vi "NI USB GPIB Command.vi"(4 "close?":bool, 6 "initialize?":bool, 8 "Error In":errorcluster, 10 "write buffer":string="X", 11 "VISA resource name":refnum<visa-resource-name>="GPIB1::25::INSTR") -> (0 "Error Out":errorcluster, 2 "read buffer":string, 3 "VISA resource name out":refnum<visa-resource-name>)   [LabVIEW 2016, in "IPS-120.lvlib"]
uses:
  IPS-120.lvlib
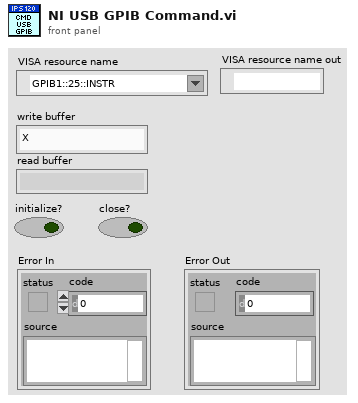
[diagram p1: front panel]
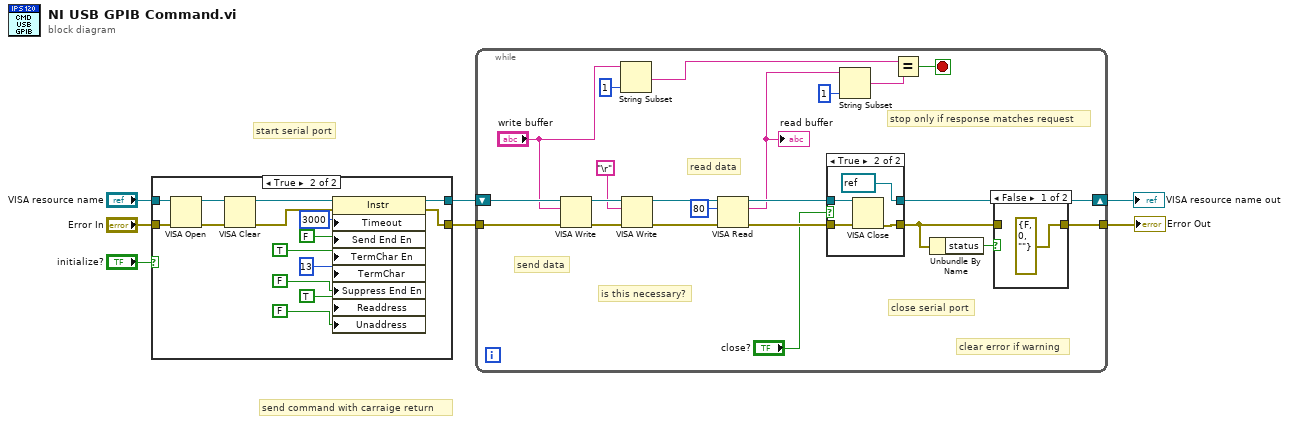
[diagram p0: block diagram]
diagram:
  # "send command with carraige return"
  # "start serial port"
  n1 = case shown="True" "initialize?" {
    tunnel: [w8 w16] -> w7
    tunnel: "Error In" -> [w9 w12]
    tunnel: [w9 w10] -> w4
    tunnel: "VISA resource name" -> [w8 w11]
    frame False {
    }
    frame True {
      n2 = VISA Open(error in (no error)=w12, VISA resource name=w11) -> (VISA resource name=w19:refnum<visa-resource-name>, error out=w20:errorcluster)  [unwired: 3 in]
      n3 = VISA Clear(VISA resource name=w19, error in (no error)=w20) -> (VISA resource name out=w17:refnum<visa-resource-name>, error out=w18:errorcluster)
      n4 = property class="Instr"(reference=w17, error in=w18, "Timeout"=u32 3000 ("General Settings:Timeout Value"), "Send End En"=FALSE ("Message Based Settings:Send End Enable"), "TermChar En"=TRUE ("Message Based Settings:Termination Character Enable"), "TermChar"=u8 13 ("Message Based Settings:Termination Character"), "Suppress End En"=FALSE ("Message Based Settings:Suppress End Enable"), "Readdress"=TRUE ("GPIB Settings:Readdressing"), "Unaddress"=FALSE ("GPIB Settings:Unaddressing")) -> (reference out=w16:refnum<visa-resource-name>, error out=w10:errorcluster)
    }
  }
  n5 = while {
    shift-right: [w28] -> w1
    shift-left: w7 -> [w42]
    tunnel: w4 -> [w34]
    tunnel: [w37] -> w6
    stop <- w25 stop-if-true
    # "stop only if response matches request"
    # "clear error if warning"
    # "is this necessary?"
    # "send data"
    # "read data"
    # "close serial port"
    n6 = VISA Write(VISA resource name=w42, write buffer="write buffer", error in (no error)=w34) -> (VISA resource name out=w40:refnum<visa-resource-name>, error out=w41:errorcluster)  [unwired: 1 out]
    n7 = String Subset(string="write buffer", length (rest)=1 ("length (rest)")) -> (substring=w26:string)  [unwired: 1 in]
    n8 = VISA Write(VISA resource name=w40, write buffer="\r", error in (no error)=w41) -> (VISA resource name out=w45:refnum<visa-resource-name>, error out=w43:errorcluster)  [unwired: 1 out]
    n9 = VISA Read(VISA resource name=w45, byte count=u32 80, error in (no error)=w43) -> (VISA resource name out=w39:refnum<visa-resource-name>, read buffer=w32:string, error out=w46:errorcluster)  [unwired: 1 out]
    "read buffer" <- w32
    n10 = case shown="True" "close?" {
      tunnel: w46 -> [w48 w52]
      tunnel: w39 -> [w47 w51]
      tunnel: [w48 w50] -> w36
      tunnel: [w47 refnum<visa-resource-name> refnum ("VISA resource name")] -> w28
      frame False {
      }
      frame True {
        n11 = VISA Close(VISA resource name=w51, error in (no error)=w52) -> (error out=w50:errorcluster)
      }
    }
    n12 = String Subset(string=w32, length (rest)=1 ("length (rest)")) -> (substring=w27:string)  [unwired: 1 in]
    n13 = Equal?(x=w26, y=w27) -> (x = y?=w25:bool)
    n14 = Unbundle By Name(w36) -> ("status"=w38:bool)
    n15 = case shown="False" w38 {
      tunnel: [errorcluster {"status"=FALSE, "code"=0, "source"=""} ("error constant") w54] -> w37
      tunnel: w36 -> [_ w54]
      frame False {
      }
      frame True {
      }
    }
  }
  "Error Out" <- w6
  "VISA resource name out" <- w1
